vi "Teleop.vi"(10 "Match Info":T1={"Autonomous Elapsed Seconds"=0.0, "TeleOp Elapsed Seconds"=0.0, "Disabled Elapsed Seconds"=0.0, "Visited Autonomous"=FALSE, "Visited TeleOp"=FALSE, "Visited Disabled"=FALSE, "Autonomous Settings"={"Autonomous Style"=enum."Independent", "VI Refnum"=refnum}}, 11 "Call Context":T2) -> ()   [LabVIEW 2012]
doc: "This VI is called for each TeleOp packet received from the DS where the robot is not disabled. It is often used to read from the joysticks and update I/O or to update setpoints for timed control loops. It should complete and return within 20 milliseconds or it may miss DS packets."
uses:
  <vilib>/Rock Robotics/WPI/DriverStation/WPI_DriverStationDerivedRobotMode.ctl
  <vilib>/Rock Robotics/WPI/DriverStation/WPI_DriverStationMatch Info.ctl
  Robot Global Data.vi
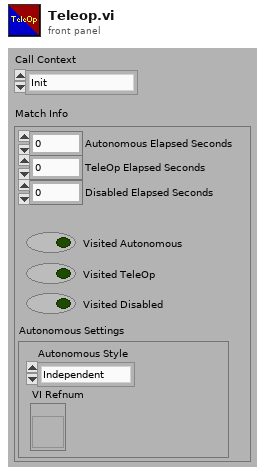
[diagram p1: front panel]
types:
  T1 = typedef "WPI_DriverStationMatch Info.ctl" = cluster{"Autonomous Elapsed Seconds":dbl, "TeleOp Elapsed Seconds":dbl, "Disabled Elapsed Seconds":dbl, "Visited Autonomous":bool, "Visited TeleOp":bool, "Visited Disabled":bool, "Autonomous Settings":cluster{"Autonomous Style":enum16{"Iterative", "Independent"}, "VI Refnum":refnum<vi>}}
  T2 = typedef "WPI_DriverStationDerivedRobotMode.ctl" = enum16{"Init", "Execute", "Stop"}
  T3 = cluster{"X":bool, "A":bool, "B":bool, "Y":bool, "LB":bool, "RB":bool, "LT":bool, "RT":bool, "Back":bool, "Start":bool, "LC":bool, "RC":bool}
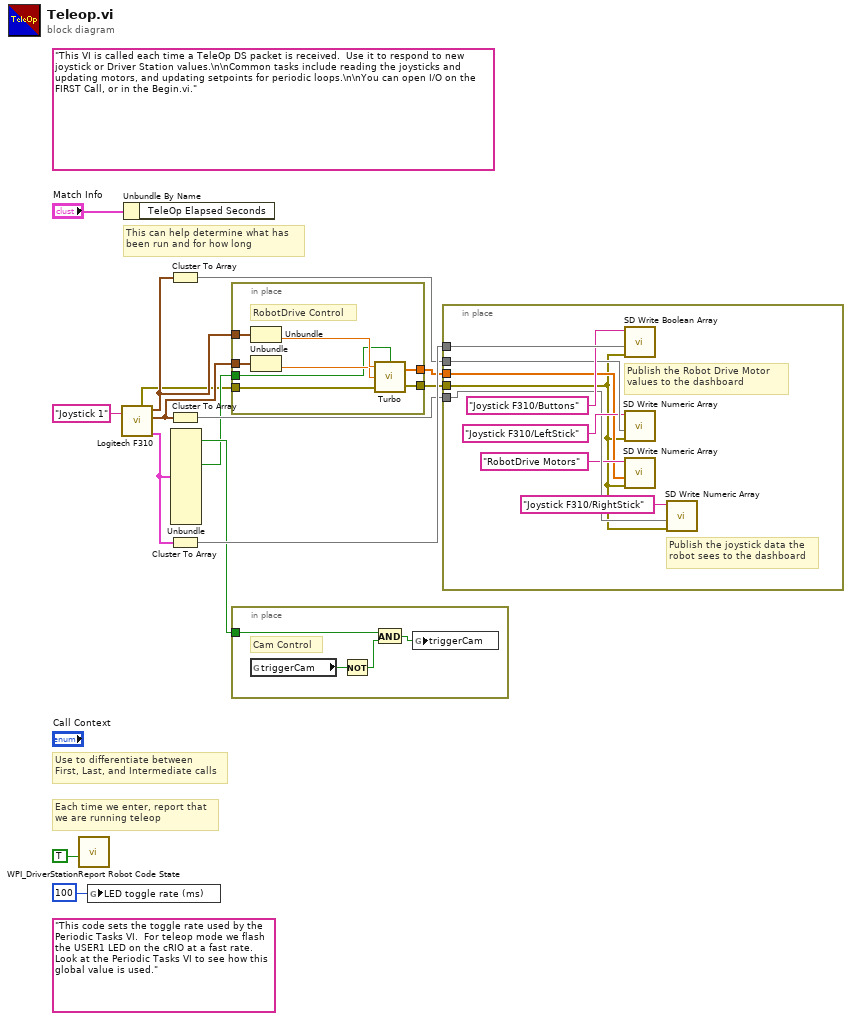
[diagram p0: block diagram]
diagram:
  (unwired) "This code sets the toggle rate used by the Periodic Tasks VI.  For teleop mode we flash the USER1 LED on the cRIO at a fast rate.  Look at the Periodic Tasks VI to see how this global value is used."
  (unwired) "This VI is called each time a TeleOp DS packet is received.  Use it to respond to new joystick or Driver Station values.\n\nCommon tasks include reading the joysticks and updating motors, and updating setpoints for periodic loops.\n\nYou can open I/O on the FIRST Call, or in the Begin.vi."
  # "Each time we enter, report that\nwe are running teleop"
  # "Use to differentiate between\nFirst, Last, and Intermediate calls"
  # "This can help determine what has\nbeen run and for how long"
  n1 = call <vilib>:"WPI_DriverStationReport Robot Code State.vi"("TeleOp"=TRUE ("Autonomous")) -> ()  [unwired: 10 in, 1 out]
  n2 = global write "Robot Global Data.vi" "LED toggle rate (ms)"(u32 100 ("LED ms toggle rate")) -> ()
  n3 = call "Logitech F310.vi"("refnum name"="Joystick 1") -> ("Buttons"=w6:T3, "Right Stick"=w7:cluster{"X":dbl, "Y":dbl}, "Left Stick"=w8:cluster{"X":dbl, "Y":dbl}, "error out"=w2:errorcluster)  [unwired: 1 in, 1 out]
  n4 = Unbundle By Name("Match Info") -> ()  [unwired: 1 out]
  n5 = Cluster To Array(cluster=w8) -> (array=w11:dbl[])
  n6 = Cluster To Array(cluster=w7) -> (array=w9:dbl[])
  n7 = Cluster To Array(cluster=w6) -> (array=w12:bool[])
  n8 = Unbundle(w6) -> ("A"=w5:bool, "LB"=w3:bool)  [unwired: 10 out]
  n9 = in-place {
    in-place-border: [w21] -> w4
    in-place-border: w8 -> [w23]
    in-place-border: w7 -> [w22]
    in-place-border: w3 -> [w18]
    in-place-border: w2 -> [w17]
    in-place-border: [w16] -> w1
    # "RobotDrive Control"
    n10 = Unbundle(w23) -> ("Y"=w20:dbl)  [unwired: 1 out]
    n11 = Unbundle(w22) -> ("Y"=w19:dbl)  [unwired: 1 out]
    n12 = call "Turbo.vi"("Turbo"=w18, "error in (no error)"=w17, "Right axis value"=w19, "Left axis value"=w20) -> ("error out"=w16:errorcluster, "Motor Values"=w21:dbl[])
  }
  n13 = in-place {
    in-place-border: w5 -> [w26]
    # "Cam Control"
    n14 = global read "Robot Global Data.vi" "triggerCam"() -> (w25:bool)
    n15 = Not(x=w25) -> (.not. x?=w27:bool)
    n16 = And(x=w26, y=w27) -> (x .and. y?=w24:bool)
    n17 = global write "Robot Global Data.vi" "triggerCam"(w24) -> ()
  }
  n18 = in-place {
    in-place-border: w12 -> [w36]
    in-place-border: w11 -> [w34]
    in-place-border: w9 -> [w31]
    in-place-border: w4 -> [w29]
    in-place-border: w1 -> [w28]
    # "Publish the joystick data the\nrobot sees to the dashboard"
    # "Publish the Robot Drive Motor\nvalues to the dashboard"
    n19 = call <vilib>:"SD Write Boolean Array.vi"("error in"=w28, "Boolean Array"=w36, "Name"="Joystick F310/Buttons") -> ()  [unwired: 7 in, 2 out]
    n20 = call <vilib>:"SD Write Numeric Array.vi"("error in"=w28, "Numeric Array"=w34, "Name"="Joystick F310/LeftStick") -> ()  [unwired: 7 in, 2 out]
    n21 = call <vilib>:"SD Write Numeric Array.vi"("error in"=w28, "Numeric Array"=w29, "Name"="RobotDrive Motors") -> ()  [unwired: 7 in, 2 out]
    n22 = call <vilib>:"SD Write Numeric Array.vi"("error in"=w28, "Numeric Array"=w31, "Name"="Joystick F310/RightStick") -> ()  [unwired: 7 in, 2 out]
  }
